vi "Make Group.vi"(11 "Array in":T1[](array[typedef])) -> (3 "Group":T7)   [LabVIEW 2020, in "Modbus Master System Explorer.lvlib"]
uses:
  Modbus Master System Explorer.lvlib
  Engine/SubVIs/Bulk Data Access.ctl
  Modbus Type.ctl
  Shared/Controls/Data Model/Channel.ctl
  <vilib>/NI VeriStand/Custom Device API/Custom Device Channel Type.ctl
  Shared/Controls/Data Model/Mapping.ctl
  Shared/Controls/Data Model/DataType.ctl
  <vilib>/NI VeriStand/Custom Device API/Custom Device Item Ref.ctl
  <vilib>/NI VeriStand/Custom Device API/Custom Device API.lvlib
  Shared/Modbus Master Shared.lvlib
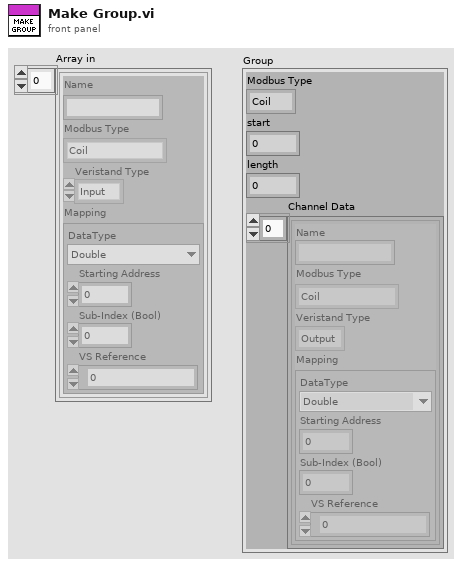
[diagram p1: front panel]
types:
  T1 = typedef "Modbus Master Shared.lvlib/Channel.ctl" = cluster{"Name":string, "Modbus Type":T2, "Veristand Type":T3, "Mapping":T4}
  T2 = typedef "Modbus Master Shared.lvlib/Modbus Type.ctl" = enum16{"Coil", "Discrete Input", "Holding Register", "Input Register"}
  T3 = typedef "Custom Device API.lvlib/Custom Device Channel Type.ctl" = enum16{"Input", "Output"}
  T4 = typedef "Modbus Master Shared.lvlib/Mapping.ctl" = cluster{"DataType":T5, "Starting Address":u16, "Sub-Index (Bool)":u16, "VS Reference":T6}
  T5 = typedef "Modbus Master Shared.lvlib/DataType.ctl" = enum16{"Double", "Single", "I64", "I32", "I16", "I8", "U64", "U32", "U16", "U8", "Boolean"}
  T6 = typedef "Custom Device API.lvlib/Custom Device Item Ref.ctl" = u64
  T7 = typedef "Modbus Master Shared.lvlib/Bulk Data Access.ctl" = cluster{"Modbus Type":T2, "start":u16, "length":u16, "Channel Data":T1[]}
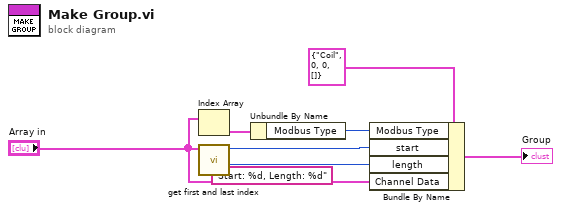
[diagram p0: block diagram]
diagram:
  (unwired) "Start: %d, Length: %d" ("format string")
  n1 = Index Array(array="Array in") -> (element=w4:T1)  [unwired: 1 in]
  n2 = call "get first and last index.vi"("Channels In"="Array in") -> ("length"=w1:u16, "Starting Register"=w2:u16)  [unwired: 8 in, 1 out]
  n3 = Unbundle By Name(w4) -> ("Modbus Type"=w5:T2)
  n4 = Bundle By Name(cluster=T7 {"Modbus Type"=enum."Coil", "start"=0, "length"=0, "Channel Data"=[]} ("output data access"), "Modbus Type"=w5, "start"=w2, "length"=w1, "Channel Data"="Array in") -> (→"Group":T7)
